vi "tcp_ip.vi"() -> ()   [LabVIEW 2020]
panel:
  in  "Slide":dbl(slide) scale=0.0..10.0
  in  "Boolean 2":bool
  in  "stop":bool
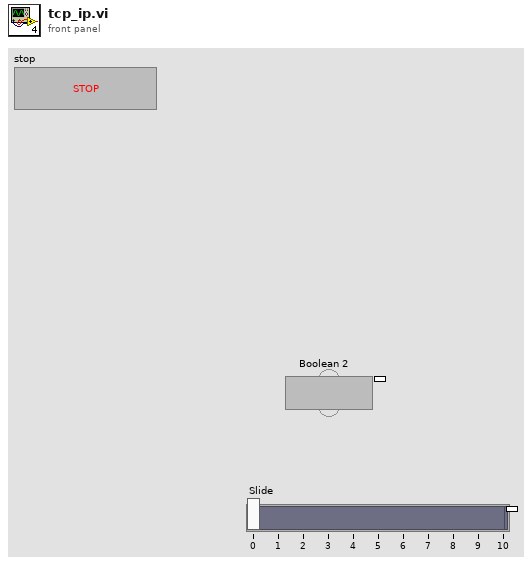
[diagram p1: front panel]
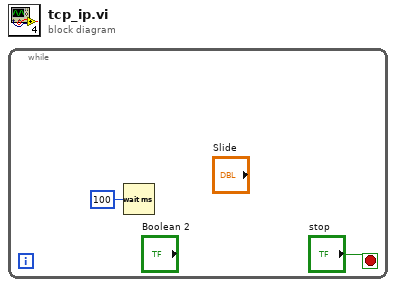
[diagram p0: block diagram]
diagram:
  n1 = while {
    stop <- "stop" stop-if-true
    n2 = Wait (ms)(milliseconds to wait=u32 100) -> ()  [unwired: 1 out]
  }
